vi "test_Timestamp (Date only).vi"(8 "error in (no error)":errorcluster, 11 "TestCase in":refnum<class "Read File Tests.lvclass">) -> (0 "error out":errorcluster, 3 "TestCase out":refnum<class "Read File Tests.lvclass">)   [LabVIEW 2017, in "Read File Tests.lvclass"]
uses:
  Read File Tests.lvclass
  Read File Tests.lvclass/Read File Tests.ctl
  Read/Read Section - Timestamp.vi
  <vilib>/addons/_JKI Toolkits/VI Tester/TestCase.llb/TestCase.lvclass
  TSC File IO.lvlib
  C:/Program Files (x86)/National Instruments/LabVIEW 2017/vi.lib/addons/_JKI Toolkits/VI Tester/TestCase.llb/TestCase.lvclass
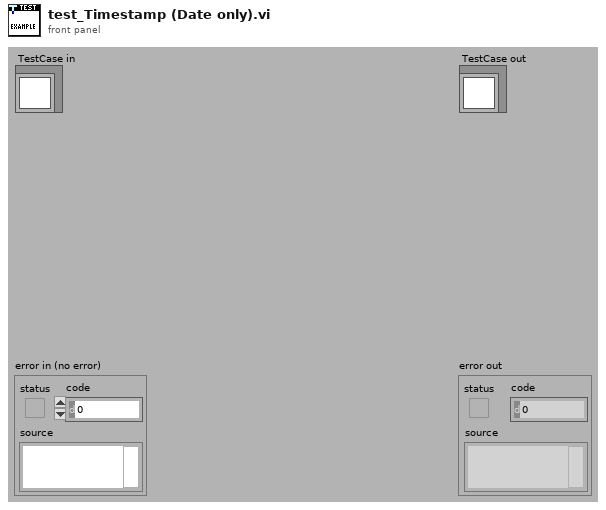
[diagram p1: front panel]
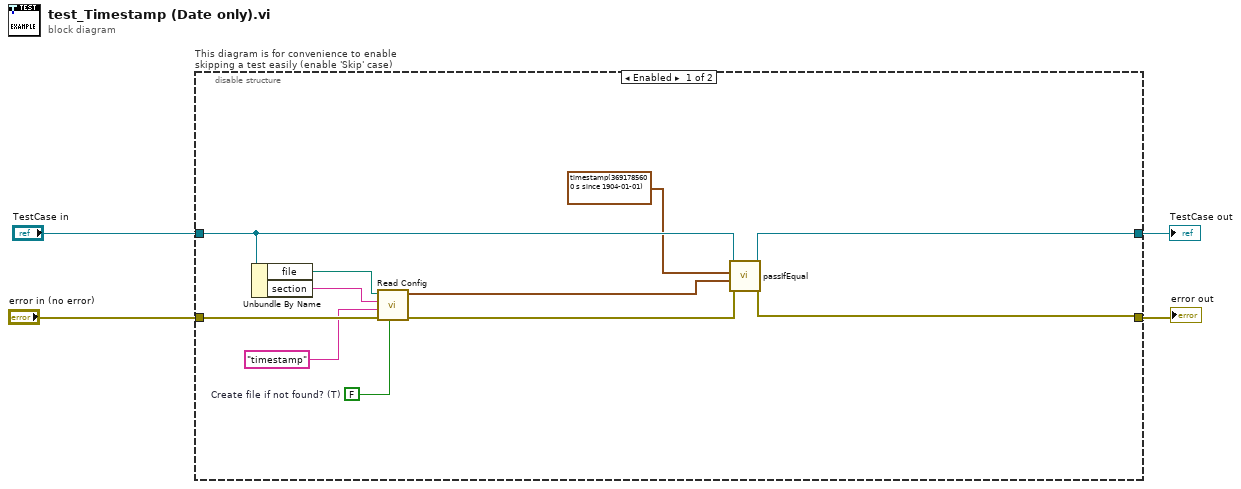
[diagram p0: block diagram]
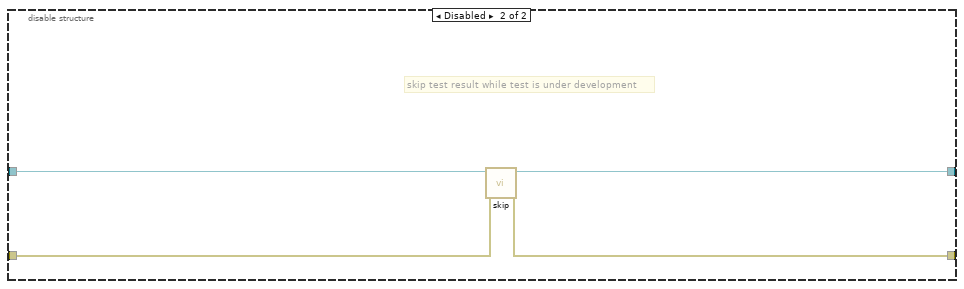
[diagram p2: hidden frame]
diagram:
  n1 = disable-structure "This diagram is for convenience to enable skipping a test easily (enable 'Skip' case)" shown="Enabled" {
    disable-tunnel: "TestCase in" -> [w13 w19]
    disable-tunnel: [w15 w17] -> w1
    disable-tunnel: [w14 w18] -> w3
    disable-tunnel: "error in (no error)" -> [w12 w16]
    frame Enabled {
      w6 = FALSE  # Create file if not found? (T)
      n2 = Unbundle By Name(w13) -> ("file"=w10:path, "section"=w9:string)
      n3 = call-poly "Read Config.vi"("Create file if not found? (T)"=w6, "error in (no error)"=w12, "key"="timestamp", "section"=w9, "Path"=w10) -> ("error out"=w11:errorcluster, "Value"=w8:timestamp)  [unwired: 5 in]
      n4 = call-dynamic "passIfEqual.vi"("error in (no error)"=w11, "y"=w8, "x"=timestamp(3691785600 s since 1904-01-01) ("Value"), "TestCase in"=w13) -> ("error out"=w14:errorcluster, "TestCase out"=w15:refnum<class "Read File Tests.lvclass">)  [unwired: 6 in]
    }
    frame Disabled {
      # "skip test result while test is under development"
      n5 = call <vilib>:"skip.vi"("error in (no error)"=w16, "TestCase in"=w19) -> ("error out"=w18:errorcluster, "TestCase out"=w17:refnum<class "Read File Tests.lvclass">)  [unwired: 8 in]
    }
  }
  "error out" <- w3
  "TestCase out" <- w1
